vi "DSF.Engine.Memory.Cache.Set Transfers.vi"(10 "Transfers":refnum<class "DSF.Engine.Transfer.lvclass">[](array[class]), 11 "Cache in":refnum<class "DSF.Engine.Memory.Cache.lvclass">) -> (3 "Cache out":refnum<class "DSF.Engine.Memory.Cache.lvclass">)   [LabVIEW 2017, in "DSF.Engine.lvlib" / "DSF.Engine.Memory.Cache.lvclass"]
uses:
  DSF.Engine.Memory.Cache.lvclass
  Transfer/DSF.Engine.Transfer.lvclass
  DSF.Engine.Memory.Cache.lvclass/DSF.Engine.Memory.Cache.ctl
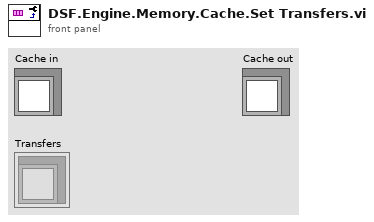
[diagram p1: front panel]
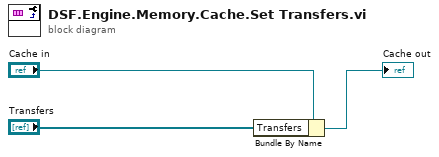
[diagram p0: block diagram]
diagram:
  n1 = Bundle By Name(cluster="Cache in", "Transfers"="Transfers") -> (→"Cache out":refnum<class "DSF.Engine.Memory.Cache.lvclass">)
